vi "2D_Jacobi_eigenvalue_algorithm_v1.vi"() -> (3 "Jacobi Eigvals":dbl[](array[numeric]))   [LabVIEW 2020]
uses:
  <vilib>/Analysis/Matrix/Datatypes/RealMatrix.ctl
  <vilib>/Analysis/7linalg.llb/Real Eigenvalues and Vectors.vi
  <vilib>/Analysis/Matrix/Numeric/Conversions/Array To Matrix - RA2.vi
  <vilib>/Analysis/baseanly.llb/Real A x B.vi
  <vilib>/Analysis/Matrix/NI_Matrix.lvlib
  <vilib>/Analysis/NI_AALBase.lvlib
  <vilib>/Analysis/NI_AALPro.lvlib
panel:
  out "summ of error":dbl
  out "LabVIEW eigvals":dbl[](array[numeric])
  out "A":T1
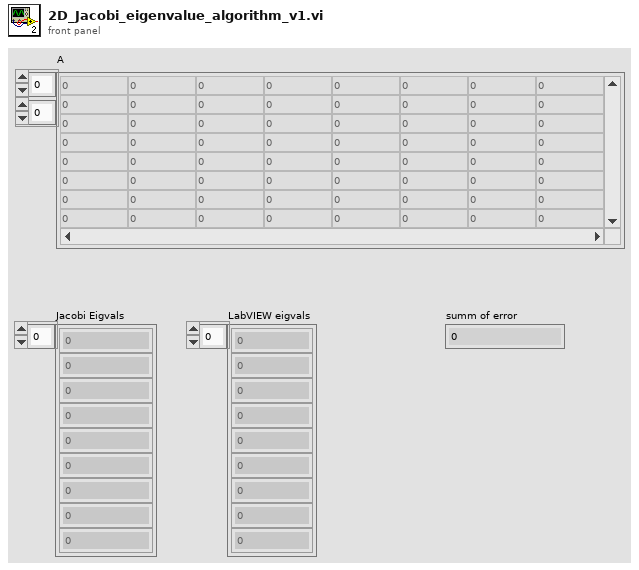
[diagram p1: front panel]
types:
  T1 = typedef "NI_Matrix.lvlib/RealMatrix.ctl" = dbl[][]
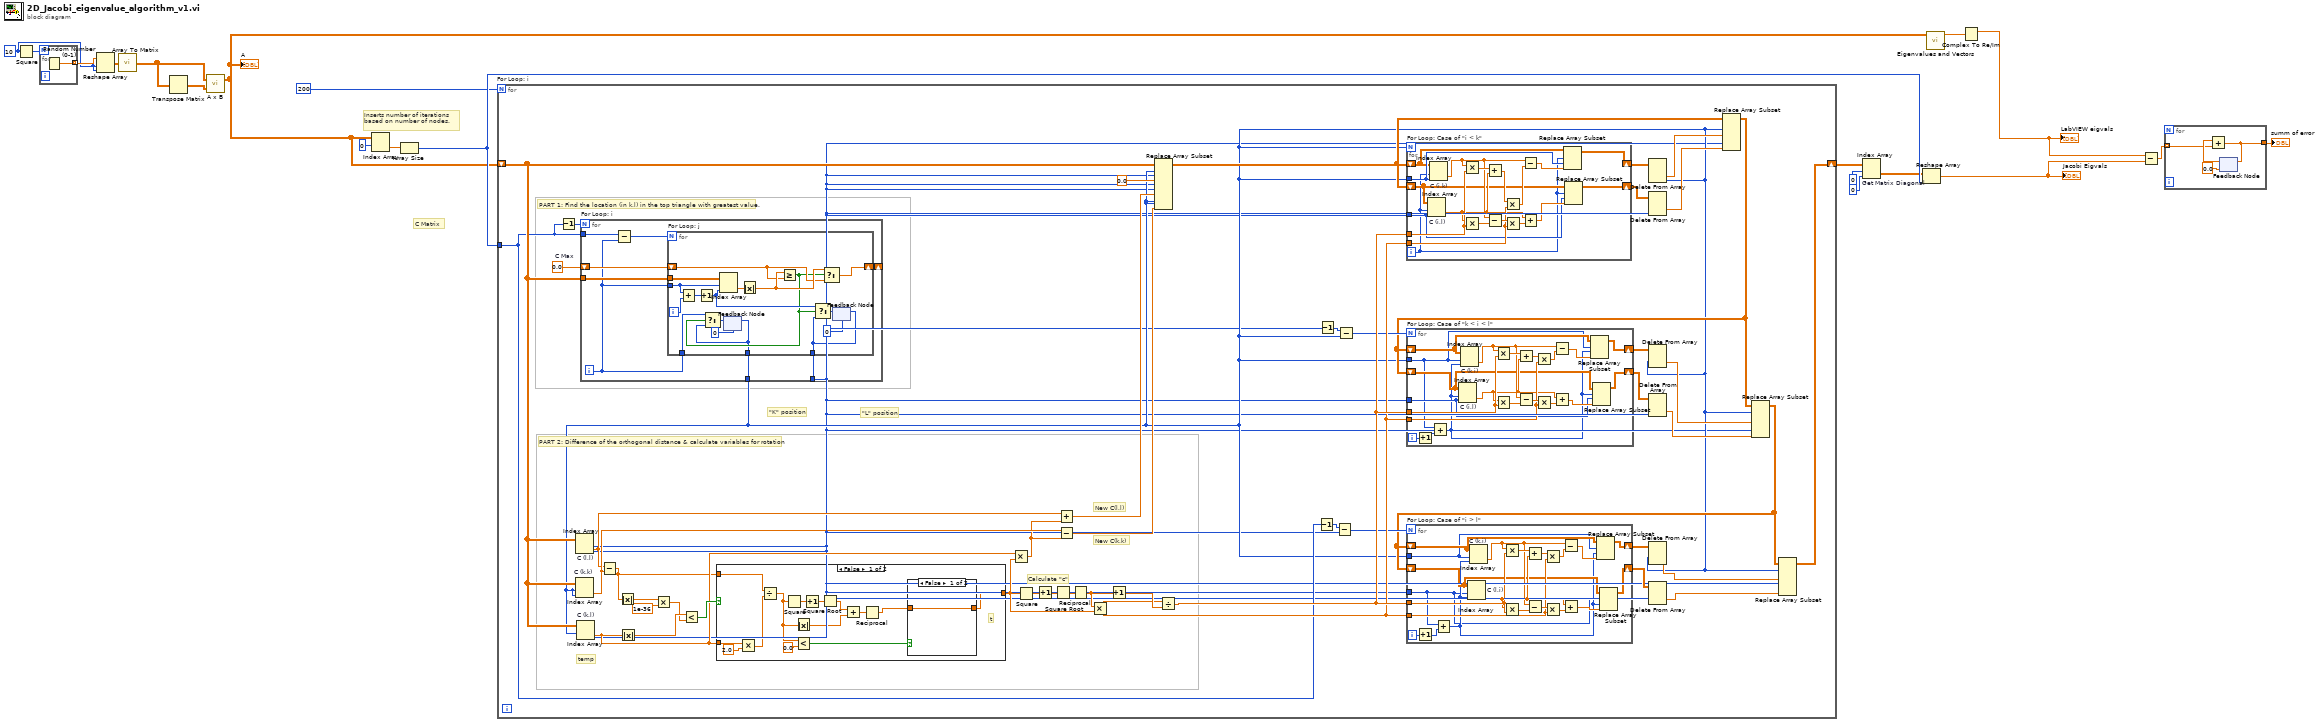
[diagram p0: block diagram]
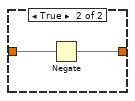
[diagram p2: hidden frame]
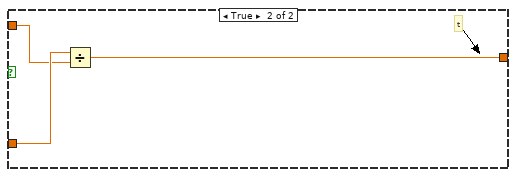
[diagram p3: hidden frame]
diagram:
  w10 = 10 ("x")
  # "C Matrix"
  # "Inserts number of iterations\nbased on number of nodes."
  n1 = Square(x=w10) -> (x^2=w12:i32)
  n2 = for {
    N: w12 -> [_]
    tunnel: [w21] -> w11 mode=indexing
    n3 = Random Number (0-1)() -> (number: 0 to 1=w21:dbl)
  }
  n4 = Reshape Array(w11, w10, w10) -> (w9:dbl[][])
  n5 = call-poly <vilib>:"Array To Matrix.vi"("Real 2D Array"=w9) -> ("Real Matrix"=w8:T1)
  n6 = Transpose Matrix(1:w8) -> (0:w7:T1)
  n7 = call-poly <vilib>:"A x B.vi"("B"=w7, "A"=w8) -> ("A x B"=w6:T1)  [unwired: 1 out]
  "A" <- w6
  n8 = Index Array(array=w6, index (row)=0) -> (element=w13:dbl[])  [unwired: 1 in]
  n9 = Array Size(array=w13) -> (size(s)=w19:i32)
  n10 = for "For Loop: i" {
    N: 200 ("Max Rotation") -> [_]
    tunnel: w19 -> [w24]
    shift-right: [w28] -> w20
    shift-left: w6 -> [w46]
    w67 = 0.0  # C Max
    # "\"L\" position"
    # "\"K\" position"
    # "PART 2: Difference of the orthogonal distance & calculate variables for rotation"
    # "PART 1: Find the location (in k,l) in the top triangle with greatest value."
    # "New C(l,l)"
    # "New C(k,k)"
    # "temp"
    # "Calculate \"c\""
    n11 = Decrement(x=w24) -> (x-1=w68:i32)
    n12 = for "For Loop: i" {
      N: w68 -> [_]
      tunnel: w46 -> [w157]
      tunnel: w24 -> [w150]
      shift-right: [w155] -> _
      shift-left: w67 -> [w153]
      tunnel: [w154] -> w22
      tunnel: [w152] -> w23
      i -> [w151]
      n13 = Subtract(x=w150, y=w151) -> (x-y=w156:i32)
      n14 = for "For Loop: j" {
        N: w156 -> [_]
        tunnel: w157 -> [w173]
        tunnel: w151 -> [w170]
        shift-right: [w167] -> w155
        shift-left: w153 -> [w168]
        tunnel: [w164] -> w154
        tunnel: [w161] -> w152
        tunnel: w151 -> [w160]
        i -> [w172]
        n15 = Add(x=w170, y=w172) -> (x+y=w171:i32)
        n16 = Increment(x=w171) -> (x+1=w166:i32)
        n17 = Index Array(array=w173, index (row)=w170, index (col)=w166) -> (element=w174:dbl)
        n18 = feedback #1(0) -> (w161:i32)
        n19 = Absolute Value(x=w174) -> (abs(x)=w169:dbl)
        n20 = Greater Or Equal?(x=w169, y=w168) -> (x >= y?=w162:bool)
        n21 = Select(t=w160, s=w162, f=w161) -> (s? t:f=w163:i32)
        n22 = feedback-in #1(w163) -> ()
        n23 = Select(t=w169, s=w162, f=w168) -> (s? t:f=w167:dbl)
        n24 = feedback #2(0) -> (w164:i32)
        n25 = Select(t=w166, s=w162, f=w164) -> (s? t:f=w165:i32)
        n26 = feedback-in #2(w165) -> ()
      }
    }
    n27 = Index Array "C (l,l)"(array=w46, index (row)=w22, index (col)=w22) -> (element=w52:dbl)
    n28 = Index Array "C (k,k)"(array=w46, index (row)=w23, index (col)=w23) -> (element=w56:dbl)
    n29 = Index Array "C (k,l)"(array=w46, index (row)=w23, index (col)=w22) -> (element=w55:dbl)
    n30 = Subtract(x=w52, y=w56) -> (x-y=w47:dbl)
    n31 = Absolute Value(x=w47) -> (abs(x)=w64:dbl)
    n32 = Absolute Value(x=w55) -> (abs(x)=w66:dbl)
    n33 = Multiply(x=w64, y=1e-36 ("x")) -> (x*y=w65:dbl)
    n34 = Less?(x=w66, y=w65) -> (x < y?=w62:bool)
    n35 = case shown="False" w62 {
      tunnel: w55 -> [w143 w149]
      tunnel: w47 -> [w140 w148]
      tunnel: [w130 w147] -> w54
      frame False {
        # "t"
        n36 = Multiply(x=w143, y=2.0) -> (x*y=w141:dbl)
        n37 = Divide(x=w140, y=w141) -> (x/y=w134:dbl)
        n38 = Square(x=w134) -> (x^2=w138:dbl)
        n39 = Absolute Value(x=w134) -> (abs(x)=w139:dbl)
        n40 = Less?(x=w134, y=0.0) -> (x < y?=w132:bool)
        n41 = Increment(x=w138) -> (x+1=w137:dbl)
        n42 = Square Root(x=w137) -> (sqrt(x)=w136:dbl)
        n43 = Add(x=w136, y=w139) -> (x+y=w135:dbl)
        n44 = Reciprocal(x=w135) -> (1/x=w131:dbl)
        n45 = case shown="False" w132 {
          tunnel: w131 -> [w144 w146]
          tunnel: [w144 w145] -> w130
          frame False {
          }
          frame True {
            n46 = Negate(x=w146) -> (-x=w145:dbl)
          }
        }
      }
      frame True {
        # "t"
        n47 = Divide(x=w149, y=w148) -> (x/y=w147:dbl)
      }
    }
    n48 = Multiply(x=w55, y=w54) -> (x*y=w53:dbl)
    n49 = Square(x=w54) -> (x^2=w61:dbl)
    n50 = Increment(x=w61) -> (x+1=w60:dbl)
    n51 = Square Root(x=w60) -> (sqrt(x)=w59:dbl)
    n52 = Add(x=w52, y=w53) -> (x+y=w44:dbl)
    n53 = Subtract(x=w56, y=w53) -> (x-y=w45:dbl)
    n54 = Reciprocal(x=w59) -> (1/x=w58:dbl)
    n55 = Multiply(x=w58, y=w54) -> (x*y=w50:dbl)
    n56 = Increment(x=w58) -> (x+1=w57:dbl)
    n57 = Replace Array Subset(array=w46, new element #1=0.0 ("new element/subarray"), index (row) #1=w23, index (col) #1=w22, new element #2=w44, index (row) #2=w22, index (col) #2=w22, new element #3=w45, index (row) #3=w23, index (col) #3=w23) -> (w39:T1)
    n58 = Divide(x=w50, y=w57) -> (x/y=w51:dbl)
    n59 = Decrement(x=w24) -> (x-1=w25:i32)
    n60 = Decrement(x=w22) -> (x-1=w26:i32)
    n61 = Subtract(x=w25, y=w22) -> (x-y=w49:i32)
    n62 = Subtract(x=w26, y=w23) -> (x-y=w48:i32)
    n63 = for "For Loop: Case of \"i < k\"" {
      N: w23 -> [_]
      tunnel: w51 -> [w126]
      tunnel: w50 -> [w123]
      tunnel: w23 -> [w118]
      tunnel: w22 -> [w113]
      shift-right: [w116] -> w43
      shift-left: w39 -> [w117]
      shift-right: [w112] -> w42
      shift-left: w39 -> [w115]
      i -> [w111]
      n64 = Index Array "C (i,l)"(array=w115, index (row)=w111, index (col)=w113) -> (element=w120:dbl)
      n65 = Index Array "C (i,k)"(array=w117, index (row)=w111, index (col)=w118) -> (element=w121:dbl)
      n66 = Multiply(x=w121, y=w126) -> (x*y=w129:dbl)
      n67 = Multiply(x=w120, y=w126) -> (x*y=w125:dbl)
      n68 = Add(x=w129, y=w120) -> (x+y=w128:dbl)
      n69 = Subtract(x=w121, y=w125) -> (x-y=w124:dbl)
      n70 = Multiply(x=w128, y=w123) -> (x*y=w127:dbl)
      n71 = Multiply(x=w124, y=w123) -> (x*y=w122:dbl)
      n72 = Subtract(x=w121, y=w127) -> (x-y=w119:dbl)
      n73 = Add(x=w120, y=w122) -> (x+y=w114:dbl)
      n74 = Replace Array Subset(array=w117, new element=w119, index (row)=w111, index (col)=w118) -> (w116:T1)
      n75 = Replace Array Subset(array=w115, new element=w114, index (row)=w111, index (col)=w113) -> (w112:T1)
    }
    n76 = Delete From Array(array=w43, index (col)=w23) -> (deleted portion=w40:dbl[])  [unwired: 2 in, 1 out]
    n77 = Delete From Array(array=w42, index (col)=w22) -> (deleted portion=w41:dbl[])  [unwired: 2 in, 1 out]
    n78 = Replace Array Subset(array=w39, new element #1=w40, index (col) #1=w23, new element #2=w41, index (col) #2=w22) -> (w36:T1)  [unwired: 2 in]
    n79 = for "For Loop: Case of \"k < i < l\"" {
      N: w48 -> [_]
      tunnel: w51 -> [w107]
      tunnel: w50 -> [w104]
      tunnel: w22 -> [w94]
      tunnel: w23 -> [w92]
      shift-right: [w98] -> w35
      shift-left: w36 -> [w100]
      shift-right: [w97] -> w34
      shift-left: w36 -> [w96]
      i -> [w91]
      n80 = Increment(x=w91) -> (x+1=w90:i32)
      n81 = Add(x=w92, y=w90) -> (x+y=w93:i32)
      n82 = Index Array "C (i,l)"(array=w96, index (row)=w93, index (col)=w94) -> (element=w101:dbl)
      n83 = Index Array "C (k,i)"(array=w100, index (row)=w92, index (col)=w93) -> (element=w102:dbl)
      n84 = Multiply(x=w102, y=w107) -> (x*y=w110:dbl)
      n85 = Multiply(x=w101, y=w107) -> (x*y=w106:dbl)
      n86 = Add(x=w110, y=w101) -> (x+y=w109:dbl)
      n87 = Subtract(x=w102, y=w106) -> (x-y=w105:dbl)
      n88 = Multiply(x=w109, y=w104) -> (x*y=w108:dbl)
      n89 = Multiply(x=w105, y=w104) -> (x*y=w103:dbl)
      n90 = Subtract(x=w102, y=w108) -> (x-y=w99:dbl)
      n91 = Add(x=w101, y=w103) -> (x+y=w95:dbl)
      n92 = Replace Array Subset(array=w100, new element=w99, index (row)=w92, index (col)=w93) -> (w98:T1)
      n93 = Replace Array Subset(array=w96, new element=w95, index (row)=w93, index (col)=w94) -> (w97:T1)
    }
    n94 = Delete From Array(array=w35, index (row)=w23) -> (deleted portion=w37:dbl[])  [unwired: 2 in, 1 out]
    n95 = Delete From Array(array=w34, index (col)=w22) -> (deleted portion=w38:dbl[])  [unwired: 2 in, 1 out]
    n96 = Replace Array Subset(array=w36, new element #1=w37, index (row) #1=w23, new element #2=w38, index (col) #2=w22) -> (w33:T1)  [unwired: 2 in]
    n97 = for "For Loop: Case of \"i > l\"" {
      N: w49 -> [_]
      tunnel: w51 -> [w86]
      tunnel: w50 -> [w83]
      tunnel: w23 -> [w77]
      tunnel: w22 -> [w71]
      shift-right: [w76] -> w32
      shift-left: w33 -> [w79]
      shift-right: [w74] -> w31
      shift-left: w33 -> [w75]
      i -> [w70]
      n98 = Increment(x=w70) -> (x+1=w69:i32)
      n99 = Add(x=w71, y=w69) -> (x+y=w72:i32)
      n100 = Index Array "C (l,i)"(array=w75, index (row)=w71, index (col)=w72) -> (element=w80:dbl)
      n101 = Index Array "C (k,i)"(array=w79, index (row)=w77, index (col)=w72) -> (element=w81:dbl)
      n102 = Multiply(x=w81, y=w86) -> (x*y=w89:dbl)
      n103 = Multiply(x=w80, y=w86) -> (x*y=w85:dbl)
      n104 = Add(x=w89, y=w80) -> (x+y=w88:dbl)
      n105 = Subtract(x=w81, y=w85) -> (x-y=w84:dbl)
      n106 = Multiply(x=w88, y=w83) -> (x*y=w87:dbl)
      n107 = Multiply(x=w84, y=w83) -> (x*y=w82:dbl)
      n108 = Subtract(x=w81, y=w87) -> (x-y=w78:dbl)
      n109 = Add(x=w80, y=w82) -> (x+y=w73:dbl)
      n110 = Replace Array Subset(array=w79, new element=w78, index (row)=w77, index (col)=w72) -> (w76:T1)
      n111 = Replace Array Subset(array=w75, new element=w73, index (row)=w71, index (col)=w72) -> (w74:T1)
    }
    n112 = Delete From Array(array=w32, index (row)=w23) -> (deleted portion=w30:dbl[])  [unwired: 2 in, 1 out]
    n113 = Delete From Array(array=w31, index (row)=w22) -> (deleted portion=w29:dbl[])  [unwired: 2 in, 1 out]
    n114 = Replace Array Subset(array=w33, new element #1=w30, index (row) #1=w23, new element #2=w29, index (row) #2=w22) -> (w28:T1)  [unwired: 2 in]
  }
  n115 = Index Array "Get Matrix Diagonal"(array=w20, index (row)=0, index (col)=0) -> (element=w17:T1)
  n116 = Reshape Array(w17, w19) -> (w3:dbl[])
  "Jacobi Eigvals" <- w3
  n117 = call-poly <vilib>:"Eigenvalues and Vectors.vi"("Input Matrix"=w6) -> ("Eigenvalues"=w5:cdb[])  [unwired: 2 in, 2 out]
  n118 = Complex To Re/Im(x + iy=w5) -> (x=w4:dbl[])  [unwired: 1 out]
  "LabVIEW eigvals" <- w4
  n119 = Subtract(x=w4, y=w3) -> (x-y=w2:dbl[])
  n120 = for {
    tunnel: w2 -> [w177] mode=indexing
    tunnel: [w175] -> w1
    n121 = feedback #3(0.0) -> (w178:dbl)
    n122 = Add(x=w178, y=w177) -> (x+y=w175:dbl)
    n123 = feedback-in #3(w175) -> ()
  }
  "summ of error" <- w1
